vi "Execute.vi"(8 "error in":errorcluster, 10 "Shifted Error in":refnum<class "Error.lvclass">, 11 "ERROR_Init in":refnum<class "ERROR_Init.lvclass">) -> (0 "error out":errorcluster, 1 "STOP?":bool, 2 "Shifted Error out":refnum<class "Error.lvclass">, 3 "ERROR_Init out":refnum<class "ERROR_Init.lvclass">)   [LabVIEW 2019, in "TSC Error.lvlib" / "ERROR_Init.lvclass"]
doc: "This Message sets original parameters for the update queue, the error log, and the location of the application's custom error code file.\n\nInputs:\n-Error in [obj] - the dynamic dispatch input class\n-Shifted Error in [obj] - the shifted error class with shared information\n-error in\n\nOutputs:\n-Error out [obj] - the dynamic dispatch output class\n-Shifted Error in [obj] - the shifted error class with shared information\n-STOP? [Boolean] - the output Boolean used to stop the Error Loop\n-error out\n\n<b>Code Developed By:</b>\nDaniel Coons\nTechnology Service Corporation\n1983 S Liberty Drive\nBloomington, IN 47403\nPhone: 812 558-7100\nwww.tsc.com\\atcs"
uses:
  ERROR_Init.lvclass
  C:/Development/Open Source/tsc-error-library/_Messages/Error/Error.lvclass
  Error/Error.lvclass
  Error/Error.lvclass/Error.ctl
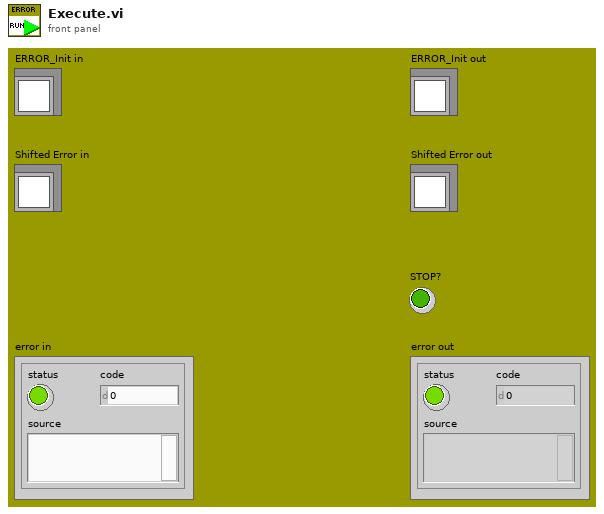
[diagram p1: front panel]
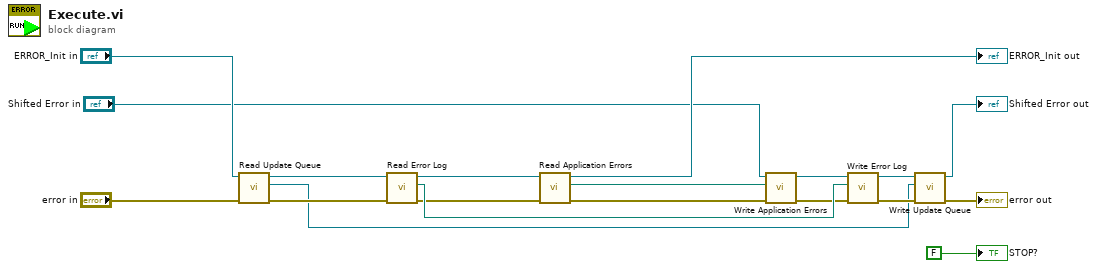
[diagram p0: block diagram]
diagram:
  n1 = call "Read Update Queue.vi"("error in (no error)"="error in", "Error in"="ERROR_Init in") -> ("error out"=w16:errorcluster, "Update Queue"=w9:refnum<queue>, "Error out"=w17:refnum<class "ERROR_Init.lvclass">)  [unwired: 7 in]
  n2 = call "Read Error Log.vi"("Error In"=w16, "Error in"=w17) -> ("Error Out"=w7:errorcluster, "Error Log"=w15:path, "Error out"=w8:refnum<class "ERROR_Init.lvclass">)  [unwired: 7 in]
  n3 = call "Read Application Errors.vi"("error in (no error)"=w7, "Error in"=w8) -> ("error out"=w5:errorcluster, "Application Errors"=w1:path, "Error out"=→"ERROR_Init out":refnum<class "ERROR_Init.lvclass">)  [unwired: 7 in]
  n4 = call "Write Application Errors.vi"("error in (no error)"=w5, "Application Errors"=w1, "Error in"="Shifted Error in") -> ("error out"=w4:errorcluster, "Error out"=w2:refnum<class "Error.lvclass">)  [unwired: 7 in]
  n5 = call "Write Error Log.vi"("error in (no error)"=w4, "Error Log"=w15, "Error in"=w2) -> ("error out"=w14:errorcluster, "Error out"=w13:refnum<class "Error.lvclass">)  [unwired: 7 in]
  n6 = call "Write Update Queue.vi"("error in (no error)"=w14, "Update Queue"=w9, "Error in"=w13) -> ("error out"=→"error out":errorcluster, "Error out"=→"Shifted Error out":refnum<class "Error.lvclass">)  [unwired: 7 in]
  "STOP?" <- FALSE ("STOP?")
